vi "Loading sci QT.vi"(0 "Absolute start time (ms)":dbl=51099.288 format="%.3f", 1 "Static input":T4(array[cluster])=[{"Times"=[6954.0, 7000.1], "Voltages"=[-0.1, -1.0], "Enable Ch"=TRUE, "Hinge Points"=2}, {"Times"=[6944.0, 6994.0, 7000.0], "Voltages"=[-1.0, 2.5, -1.0], "Enable Ch"=TRUE, "Hinge Points"=3}, {"Times"=[6944.0, 6994.0, 7000.0], "Voltages"=[0.0, 0.6, -1.0], "Enable Ch"=TRUE, "Hinge Points"=3}, {"Times"=[6944.0, 6994.0, 7000.0], "Voltages"=[4.0, 0.65, -1.0], "Enable Ch"=TRUE, "Hinge Points"=3}, {"Times"=[6992.0, 7000.6], "Voltages"=[0.0, 2.7], "Enable Ch"=TRUE, "Hinge Points"=2}, {"Times"=[7000.6, 7011.1], "Voltages"=[0.25, 3.0], "Enable Ch"=TRUE, "Hinge Points"=2}, {"Times"=[], "Voltages"=[], "Enable Ch"=TRUE, "Hinge Points"=0}, {"Times"=[48001.288, 48011.488, 48021.688, 48031.888, 48042.088, 48052.288, 48062.488, 48072.688, 48082.888, 48093.088, 48103.288, 48113.488, 48123.688, 48133.888, 48144.088, 48154.288, 48164.488, 48174.688, 48184.888, 48195.088, 48205.288, 48215.488, 48225.688, 48235.888, 48246.088, 48256.288, 48266.488, 48276.688, 48286.888, 48297.088, 48307.288, 48317.488, 48327.688, 48337.888, 48348.088, 48358.288, 48368.488, 48378.688, 48388.888, 48399.088, 48409.288, 48419.488, 48429.688, 48439.888, 48450.088, 48460.288, 48470.488, 48480.688, 48490.888, 48501.088, 48511.288], "Voltages"=[0.0, -0.0052, -0.0104, -0.0156, -0.0208, -0.026, -0.0312, -0.0364, -0.0416, -0.046799999999999994, -0.052, -0.0572, -0.0624, -0.0676, -0.0728, -0.078, -0.0832, -0.08839999999999999, -0.09359999999999999, -0.0988, -0.104, -0.10919999999999999, -0.1144, -0.1196, -0.1248, -0.13, -0.1352, -0.1404, -0.1456, -0.1508, -0.156, -0.16119999999999998, -0.1664, -0.1716, -0.17679999999999998, -0.182, -0.18719999999999998, -0.1924, -0.1976, -0.20279999999999998, -0.208, -0.2132, -0.21839999999999998, -0.2236, -0.2288, -0.23399999999999999, -0.2392, -0.24439999999999998, -0.2496, -0.25479999999999997, -0.26], "Enable Ch"=TRUE, "Hinge Points"=51}, {"Times"=[6944.0, 6994.0, 7000.1, 7004.1, 47301.288, 47631.288, 50900.288, 51105.288], "Voltages"=[0.1635, 0.12, -0.63, 0.0, 0.067, -0.004, 1.44, -0.004], "Enable Ch"=TRUE, "Hinge Points"=8}, {"Times"=[6994.0, 7000.0, 7001.0, 7003.1, 7103.1, 7105.6, 7108.1, 7110.6, 7113.1, 7115.6, 7118.1, 7120.6, 7123.1, 7125.6, 7128.1, 7130.6, 7133.1, 7135.6, 7138.1, 7140.6, 7143.1, 7145.6, 7148.1, 7150.6, 7153.1, 7155.6, 7158.1, 7160.6, 7163.1, 7165.6, 7168.1, 7170.6, 7173.1, 7175.6, 7178.1, 7180.6, 7183.1, 7185.6, 7188.1, 7190.6, 7193.1, 7195.6, 7198.1, 7200.6, 7203.1, 7205.6, 7208.1, 7210.6, 7213.1, 7215.6, 7218.1, 7220.6, 7223.1, 7225.6, 7228.1, 7230.6, 7233.1, 7235.6, 7238.1, 7240.6, 7243.1, 7245.6, 7248.1, 7250.6, 7253.1, 7255.6, 7258.1, 7260.6, 7263.1, 7265.6, 7268.1, 7270.6, 7273.1, 7275.6, 7278.1, 7280.6, 7283.1, 7285.6, 7288.1, 7290.6, 7293.1, 7295.6, 7298.1, 7300.6, 7303.1, 7305.6, 7308.1, 7310.6, 7313.1, 7315.6, 7318.1, 7320.6, 7323.1, 7325.6, 7328.1, 7330.6, 7333.1, 7335.6, 7338.1, 7340.6, 7343.1, 7345.6, 7348.1, 7350.6, 7353.1, 10849.9], "Voltages"=[-1.0, -10.0, 0.0, 1.8, 1.8, 1.854, 1.9080000000000001, 1.9620000000000002, 2.016, 2.0700000000000003, 2.124, 2.178, 2.232, 2.286, 2.34, 2.394, 2.4480000000000004, 2.5020000000000002, 2.556, 2.6100000000000003, 2.664, 2.718, 2.7720000000000002, 2.826, 2.88, 2.934, 2.9880000000000004, 3.0420000000000003, 3.096, 3.1500000000000004, 3.204, 3.258, 3.3120000000000003, 3.3660000000000005, 3.42, 3.474, 3.5280000000000005, 3.5820000000000003, 3.636, 3.6900000000000004, 3.744, 3.798, 3.8520000000000003, 3.9060000000000006, 3.96, 4.014, 4.0680000000000005, 4.122, 4.176, 4.23, 4.284000000000001, 4.338, 4.392, 4.446000000000001, 4.5, 4.554, 4.6080000000000005, 4.662000000000001, 4.716, 4.7700000000000005, 4.824000000000001, 4.878, 4.932, 4.986000000000001, 5.04, 5.094, 5.148000000000001, 5.202000000000001, 5.256, 5.3100000000000005, 5.364000000000001, 5.418, 5.472, 5.526000000000001, 5.58, 5.634, 5.688000000000001, 5.742000000000001, 5.796, 5.8500000000000005, 5.904, 5.958, 6.0120000000000005, 6.066000000000001, 6.12, 6.174, 6.228000000000001, 6.282, 6.336, 6.390000000000001, 6.444, 6.498, 6.5520000000000005, 6.606000000000001, 6.66, 6.714, 6.768000000000001, 6.822, 6.876, 6.930000000000001, 6.984000000000001, 7.038, 7.0920000000000005, 7.146000000000001, 7.2, -1.0], "Enable Ch"=TRUE, "Hinge Points"=106}, {"Times"=[7001.0, 6978.1, 7008.1, 7093.1, 7095.6, 7098.1, 7100.6, 7103.1, 7105.6, 7108.1, 7110.6, 7113.1, 7115.6, 7118.1, 7120.6, 7123.1, 7125.6, 7128.1, 7130.6, 7133.1, 7135.6, 7138.1, 7140.6, 7143.1, 7145.6, 7148.1, 7150.6, 7153.1, 7155.6, 7158.1, 7160.6, 7163.1, 7165.6, 7168.1, 7170.6, 7173.1, 7175.6, 7178.1, 7180.6, 7183.1, 7185.6, 7188.1, 7190.6, 7193.1, 7195.6, 7198.1, 7200.6, 7203.1, 7205.6, 7208.1, 7210.6, 7213.1, 7215.6, 7218.1, 7220.6, 7223.1, 7225.6, 7228.1, 7230.6, 7233.1, 7235.6, 7238.1, 7240.6, 7243.1, 7245.6, 7248.1, 7250.6, 7253.1, 7255.6, 7258.1, 7260.6, 7263.1, 7265.6, 7268.1, 7270.6, 7273.1, 7275.6, 7278.1, 7280.6, 7283.1, 7285.6, 7288.1, 7290.6, 7293.1, 7295.6, 7298.1, 7300.6, 7303.1, 7305.6, 7308.1, 7310.6, 7313.1, 7315.6, 7318.1, 7320.6, 7323.1, 7325.6, 7328.1, 7330.6, 7333.1, 7335.6, 7338.1, 7340.6, 7343.1, 10855.0, 47201.288, 47206.288, 47951.288, 48101.788, 48471.288], "Voltages"=[-0.4, -2.5, -0.78, -0.78, -0.8009000000000001, -0.8218, -0.8427, -0.8636, -0.8845000000000001, -0.9054, -0.9263, -0.9472, -0.9681, -0.989, -1.0099, -1.0308, -1.0517, -1.0726, -1.0935000000000001, -1.1144, -1.1353, -1.1562000000000001, -1.1771, -1.198, -1.2189, -1.2398, -1.2607, -1.2816, -1.3025, -1.3234, -1.3443, -1.3652, -1.3860999999999999, -1.407, -1.4279, -1.4487999999999999, -1.4697, -1.4906, -1.5114999999999998, -1.5324, -1.5533000000000001, -1.5741999999999998, -1.5951, -1.616, -1.6368999999999998, -1.6578, -1.6787, -1.6996, -1.7205, -1.7414, -1.7623, -1.7832, -1.8041, -1.825, -1.8458999999999999, -1.8668, -1.8877, -1.9085999999999999, -1.9295, -1.9504, -1.9712999999999998, -1.9922, -2.0130999999999997, -2.034, -2.0549, -2.0758, -2.0967000000000002, -2.1176, -2.1384999999999996, -2.1593999999999998, -2.1803, -2.2012, -2.2221, -2.243, -2.2639, -2.2847999999999997, -2.3057, -2.3266, -2.3475, -2.3684, -2.3893, -2.4101999999999997, -2.4311, -2.452, -2.4729, -2.4938, -2.5147, -2.5355999999999996, -2.5564999999999998, -2.5774, -2.5983, -2.6192, -2.6401, -2.6609999999999996, -2.6818999999999997, -2.7028, -2.7237, -2.7446, -2.7655, -2.7863999999999995, -2.8072999999999997, -2.8282, -2.8491, -2.87, -1.52, -0.5, -0.15, -2.0, -1.8, -2.4], "Enable Ch"=TRUE, "Hinge Points"=110}, {"Times"=[6944.0, 6994.0, 7000.6], "Voltages"=[0.15, 0.2, 2.5], "Enable Ch"=TRUE, "Hinge Points"=3}, {"Times"=[10850.0, 47200.188, 47200.288, 47200.338, 47200.388, 47200.438, 47200.488, 47200.538, 47200.588, 47200.638, 47200.688, 47200.738, 47200.788, 47200.838, 47200.888, 47200.938, 47200.988, 47201.038, 47201.088, 47201.138, 47201.188, 47201.238, 47201.288, 48501.788, 48001.288, 48003.788, 48006.288, 48008.788, 48011.288, 48013.788, 48016.288, 48018.788, 48021.288, 48023.788, 48026.288, 48028.788, 48031.288, 48033.788, 48036.288, 48038.788, 48041.288, 48043.788, 48046.288, 48048.788, 48051.288, 48053.788, 48056.288, 48058.788, 48061.288, 48063.788, 48066.288, 48068.788, 48071.288, 48073.788, 48076.288, 48078.788, 48081.288, 48083.788, 48086.288, 48088.788, 48091.288, 48093.788, 48096.288, 48098.788, 48101.288, 48103.788, 48106.288, 48108.788, 48111.288, 48113.788, 48116.288, 48118.788, 48121.288, 48123.788, 48126.288, 48128.788, 48131.288, 48133.788, 48136.288, 48138.788, 48141.288, 48143.788, 48146.288, 48148.788, 48151.288, 48153.788, 48156.288, 48158.788, 48161.288, 48163.788, 48166.288, 48168.788, 48171.288, 48173.788, 48176.288, 48178.788, 48181.288, 48183.788, 48186.288, 48188.788, 48191.288, 48193.788, 48196.288, 48198.788, 48201.288, 48203.788, 48206.288, 48208.788, 48211.288, 48213.788, 48216.288, 48218.788, 48221.288, 48223.788, 48226.288, 48228.788, 48231.288, 48233.788, 48236.288, 48238.788, 48241.288, 48243.788, 48246.288, 48248.788, 48251.288, 48253.788, 48256.288, 48258.788, 48261.288, 48263.788, 48266.288, 48268.788, 48271.288, 48273.788, 48276.288, 48278.788, 48281.288, 48283.788, 48286.288, 48288.788, 48291.288, 48293.788, 48296.288, 48298.788, 48301.288, 48303.788, 48306.288, 48308.788, 48311.288, 48313.788, 48316.288, 48318.788, 48321.288, 48323.788, 48326.288, 48328.788, 48331.288, 48333.788, 48336.288, 48338.788, 48341.288, 48343.788, 48346.288, 48348.788, 48351.288, 48353.788, 48356.288, 48358.788, 48361.288, 48363.788, 48366.288, 48368.788, 48371.288, 48373.788, 48376.288, 48378.788, 48381.288, 48383.788, 48386.288, 48388.788, 48391.288, 48393.788, 48396.288, 48398.788, 48401.288, 48403.788, 48406.288, 48408.788, 48411.288, 48413.788, 48416.288, 48418.788, 48421.288, 48423.788, 48426.288, 48428.788, 48431.288, 48433.788, 48436.288, 48438.788, 48441.288, 48443.788, 48446.288, 48448.788, 48451.288, 48453.788, 48456.288, 48458.788, 48461.288, 48463.788, 48466.288, 48468.788, 48471.288, 48473.788, 48476.288, 48478.788, 48481.288, 48483.788, 48486.288, 48488.788, 48491.288, 48493.788, 48496.288, 48498.788, 48501.288], "Voltages"=[0.0, 2.978, 2.978, 2.8241, 2.6702000000000004, 2.5163, 2.3624, 2.2085, 2.0546, 1.9007, 1.7468000000000001, 1.5929000000000002, 1.439, 1.2851000000000001, 1.1312000000000002, 0.9773000000000001, 0.8233999999999999, 0.6695000000000002, 0.5156000000000001, 0.3616999999999999, 0.2078000000000002, 0.05390000000000006, -0.10000000000000009, 0.0, 0.0, 0.00065, 0.0013, 0.00195, 0.0026, 0.00325, 0.0039, 0.00455, 0.0052, 0.005849999999999999, 0.0065, 0.00715, 0.0078, 0.00845, 0.0091, 0.00975, 0.0104, 0.011049999999999999, 0.011699999999999999, 0.01235, 0.013, 0.013649999999999999, 0.0143, 0.01495, 0.0156, 0.01625, 0.0169, 0.01755, 0.0182, 0.01885, 0.0195, 0.020149999999999998, 0.0208, 0.02145, 0.022099999999999998, 0.02275, 0.023399999999999997, 0.02405, 0.0247, 0.025349999999999998, 0.026, 0.02665, 0.027299999999999998, 0.02795, 0.0286, 0.029249999999999998, 0.0299, 0.030549999999999997, 0.0312, 0.031849999999999996, 0.0325, 0.03315, 0.0338, 0.03445, 0.0351, 0.03575, 0.0364, 0.03705, 0.0377, 0.038349999999999995, 0.039, 0.03965, 0.040299999999999996, 0.04095, 0.0416, 0.042249999999999996, 0.0429, 0.04355, 0.044199999999999996, 0.04485, 0.0455, 0.04615, 0.046799999999999994, 0.04745, 0.0481, 0.048749999999999995, 0.0494, 0.05005, 0.050699999999999995, 0.05135, 0.052, 0.052649999999999995, 0.0533, 0.05395, 0.054599999999999996, 0.05525, 0.0559, 0.056549999999999996, 0.0572, 0.05785, 0.058499999999999996, 0.059149999999999994, 0.0598, 0.06045, 0.061099999999999995, 0.06175, 0.0624, 0.06305, 0.06369999999999999, 0.06434999999999999, 0.065, 0.06565, 0.0663, 0.06695, 0.0676, 0.06824999999999999, 0.0689, 0.06955, 0.0702, 0.07085, 0.0715, 0.07214999999999999, 0.0728, 0.07345, 0.0741, 0.07475, 0.0754, 0.07604999999999999, 0.07669999999999999, 0.07735, 0.078, 0.07865, 0.0793, 0.07995, 0.08059999999999999, 0.08125, 0.0819, 0.08255, 0.0832, 0.08385, 0.08449999999999999, 0.08514999999999999, 0.0858, 0.08645, 0.0871, 0.08775, 0.08839999999999999, 0.08904999999999999, 0.0897, 0.09035, 0.091, 0.09165, 0.0923, 0.09294999999999999, 0.09359999999999999, 0.09425, 0.0949, 0.09555, 0.0962, 0.09684999999999999, 0.09749999999999999, 0.09815, 0.0988, 0.09945, 0.1001, 0.10074999999999999, 0.10139999999999999, 0.10205, 0.1027, 0.10335, 0.104, 0.10464999999999999, 0.10529999999999999, 0.10594999999999999, 0.1066, 0.10725, 0.1079, 0.10855, 0.10919999999999999, 0.10984999999999999, 0.1105, 0.11115, 0.1118, 0.11245, 0.11309999999999999, 0.11374999999999999, 0.1144, 0.11505, 0.1157, 0.11635, 0.11699999999999999, 0.11764999999999999, 0.11829999999999999, 0.11895, 0.1196, 0.12025, 0.1209, 0.12154999999999999, 0.12219999999999999, 0.12285, 0.1235, 0.12415, 0.1248, 0.12545, 0.1261, 0.12675, 0.12739999999999999, 0.12805, 0.12869999999999998, 0.12935, 0.13], "Enable Ch"=TRUE, "Hinge Points"=225}, {"Times"=[10850.0, 10950.0, 10959.0, 10968.0, 10977.0, 10986.0, 10995.0, 11004.0, 11013.0, 11022.0, 11031.0, 11040.0, 11049.0, 11058.0, 11067.0, 11076.0, 11085.0, 11094.0, 11103.0, 11112.0, 11121.0, 11130.0, 11139.0, 11148.0, 11157.0, 11166.0, 11175.0, 11184.0, 11193.0, 11202.0, 11211.0, 11220.0, 11229.0, 11238.0, 11247.0, 11256.0, 11265.0, 11274.0, 11283.0, 11292.0, 11301.0, 11310.0, 11319.0, 11328.0, 11337.0, 11346.0, 11355.0, 11364.0, 11373.0, 11382.0, 11391.0, 11400.0, 11409.0, 11418.0, 11427.0, 11436.0, 11445.0, 11454.0, 11463.0, 11472.0, 11481.0, 11490.0, 11499.0, 11508.0, 11517.0, 11526.0, 11535.0, 11544.0, 11553.0, 11562.0, 11571.0, 11580.0, 11589.0, 11598.0, 11607.0, 11616.0, 11625.0, 11634.0, 11643.0, 11652.0, 11661.0, 11670.0, 11679.0, 11688.0, 11697.0, 11706.0, 11715.0, 11724.0, 11733.0, 11742.0, 11751.0, 11760.0, 11769.0, 11778.0, 11787.0, 11796.0, 11805.0, 11814.0, 11823.0, 11832.0, 11841.0, 11850.0, 47191.188, 47200.288, 47205.288, 47201.288, 47201.338, 47201.388, 47201.438, 47201.488, 47201.538, 47201.588, 47201.638, 47201.688, 47201.738, 47201.788, 47201.838, 47201.888, 47201.938, 47201.988, 47202.038, 47202.088, 47202.138, 47202.188, 47202.238, 47202.288, 47202.338, 47202.388, 47202.438, 47202.488, 47202.538, 47202.588, 47202.638, 47202.688, 47202.738, 47202.788, 47202.838, 47202.888, 47202.938, 47202.988, 47203.038, 47203.088, 47203.138, 47203.188, 47203.238, 47203.288, 47203.338, 47203.388, 47203.438, 47203.488, 47203.538, 47203.588, 47203.638, 47203.688, 47203.738, 47203.788, 47203.838, 47203.888, 47203.938, 47203.988, 47204.038, 47204.088, 47204.138, 47204.188, 47204.238, 47204.288, 47191.288, 47191.348, 47191.408, 47191.468, 47191.528, 47191.588, 47191.648, 47191.708, 47191.768000000004, 47191.828, 47191.888, 47191.948000000004, 47192.008, 47192.068, 47192.128, 47192.188, 47192.248, 47192.308, 47192.368, 47192.428, 47192.488, 47192.548, 47192.608, 47192.668, 47192.728, 47192.788, 47192.848, 47192.908, 47192.968, 47193.028, 47193.088, 47193.148, 47193.208, 47193.268000000004, 47193.328, 47193.388, 47193.448000000004, 47193.508, 47193.568, 47193.628, 47193.688, 47193.748, 47193.808, 47193.868, 47193.928, 47193.988, 47194.048, 47194.108, 47194.168, 47194.228, 47194.288, 47194.348, 47194.408, 47194.468, 47194.528, 47194.588, 47194.648, 47194.708, 47194.768000000004, 47194.828, 47194.888, 47194.948000000004, 47195.008, 47195.068, 47195.128, 47195.188, 47195.248, 47195.308, 47195.368, 47195.428, 47195.488, 47195.548, 47195.608, 47195.668, 47195.728, 47195.788, 47195.848, 47195.908, 47195.968, 47196.028, 47196.088, 47196.148, 47196.208, 47196.268000000004, 47196.328, 47196.388, 47196.448000000004, 47196.508, 47196.568, 47196.628, 47196.688, 47196.748, 47196.808, 47196.868, 47196.928, 47196.988, 47197.048, 47197.108, 47197.168, 47197.228, 47197.288, 47501.288, 47501.288, 47501.368, 47501.448000000004, 47501.528, 47501.608, 47501.688, 47501.768000000004, 47501.848, 47501.928, 47502.008, 47502.088, 47502.168, 47502.248, 47502.328, 47502.408, 47502.488, 47502.568, 47502.648, 47502.728, 47502.808, 47502.888, 47502.968, 47503.048, 47503.128, 47503.208, 47503.288, 47503.368, 47503.448000000004, 47503.528, 47503.608, 47503.688, 47503.768000000004, 47503.848, 47503.928, 47504.008, 47504.088, 47504.168, 47504.248, 47504.328, 47504.408, 47504.488, 47504.568, 47504.648, 47504.728, 47504.808, 47504.888, 47504.968, 47505.048, 47505.128, 47505.208, 47505.288, 48511.788, 48001.288, 48003.788, 48006.288, 48008.788, 48011.288, 48013.788, 48016.288, 48018.788, 48021.288, 48023.788, 48026.288, 48028.788, 48031.288, 48033.788, 48036.288, 48038.788, 48041.288, 48043.788, 48046.288, 48048.788, 48051.288, 48053.788, 48056.288, 48058.788, 48061.288, 48063.788, 48066.288, 48068.788, 48071.288, 48073.788, 48076.288, 48078.788, 48081.288, 48083.788, 48086.288, 48088.788, 48091.288, 48093.788, 48096.288, 48098.788, 48101.288, 48103.788, 48106.288, 48108.788, 48111.288, 48113.788, 48116.288, 48118.788, 48121.288, 48123.788, 48126.288, 48128.788, 48131.288, 48133.788, 48136.288, 48138.788, 48141.288, 48143.788, 48146.288, 48148.788, 48151.288, 48153.788, 48156.288, 48158.788, 48161.288, 48163.788, 48166.288, 48168.788, 48171.288, 48173.788, 48176.288, 48178.788, 48181.288, 48183.788, 48186.288, 48188.788, 48191.288, 48193.788, 48196.288, 48198.788, 48201.288, 48203.788, 48206.288, 48208.788, 48211.288, 48213.788, 48216.288, 48218.788, 48221.288, 48223.788, 48226.288, 48228.788, 48231.288, 48233.788, 48236.288, 48238.788, 48241.288, 48243.788, 48246.288, 48248.788, 48251.288, 48253.788, 48256.288, 48258.788, 48261.288, 48263.788, 48266.288, 48268.788, 48271.288, 48273.788, 48276.288, 48278.788, 48281.288, 48283.788, 48286.288, 48288.788, 48291.288, 48293.788, 48296.288, 48298.788, 48301.288, 48303.788, 48306.288, 48308.788, 48311.288, 48313.788, 48316.288, 48318.788, 48321.288, 48323.788, 48326.288, 48328.788, 48331.288, 48333.788, 48336.288, 48338.788, 48341.288, 48343.788, 48346.288, 48348.788, 48351.288, 48353.788, 48356.288, 48358.788, 48361.288, 48363.788, 48366.288, 48368.788, 48371.288, 48373.788, 48376.288, 48378.788, 48381.288, 48383.788, 48386.288, 48388.788, 48391.288, 48393.788, 48396.288, 48398.788, 48401.288, 48403.788, 48406.288, 48408.788, 48411.288, 48413.788, 48416.288, 48418.788, 48421.288, 48423.788, 48426.288, 48428.788, 48431.288, 48433.788, 48436.288, 48438.788, 48441.288, 48443.788, 48446.288, 48448.788, 48451.288, 48453.788, 48456.288, 48458.788, 48461.288, 48463.788, 48466.288, 48468.788, 48471.288, 48473.788, 48476.288, 48478.788, 48481.288, 48483.788, 48486.288, 48488.788, 48491.288, 48493.788, 48496.288, 48498.788, 48501.288, 48501.288, 48502.288, 48503.288, 48504.288, 48505.288, 48506.288, 48507.288, 48508.288, 48509.288, 48510.288, 48511.288, 50899.288, 50904.288, 50909.288, 50914.288, 50919.288, 50924.288, 50929.288, 50934.288, 50939.288, 50944.288, 50949.288, 50954.288, 50959.288, 50964.288, 50969.288, 50974.288, 50979.288, 50984.288, 50989.288, 50994.288, 50999.288, 51098.288, 51098.29466666667, 51098.30133333334, 51098.308, 51098.314666666665, 51098.32133333333, 51098.328, 51098.33466666667, 51098.34133333334, 51098.348, 51098.354666666666, 51098.361333333334, 51098.368, 51098.37466666667, 51098.38133333333, 51098.388, 51098.39466666667, 51098.401333333335, 51098.408, 51098.414666666664, 51098.42133333333, 51098.428, 51098.43466666667, 51098.441333333336, 51098.448000000004, 51098.454666666665, 51098.46133333333, 51098.468, 51098.47466666667, 51098.48133333334, 51098.488, 51098.494666666666, 51098.50133333333, 51098.508, 51098.51466666667, 51098.52133333333, 51098.528, 51098.53466666667, 51098.541333333334, 51098.548, 51098.55466666667, 51098.56133333333, 51098.568, 51098.57466666667, 51098.581333333335, 51098.588, 51098.594666666664, 51098.60133333333, 51098.608, 51098.61466666667, 51098.621333333336, 51098.628, 51098.634666666665, 51098.64133333333, 51098.648, 51098.65466666667, 51098.66133333334, 51098.668, 51098.674666666666, 51098.681333333334, 51098.688, 51098.69466666667, 51098.70133333333, 51098.708, 51098.71466666667, 51098.721333333335, 51098.728, 51098.73466666666, 51098.74133333333, 51098.748, 51098.75466666667, 51098.761333333336, 51098.768000000004, 51098.774666666664, 51098.78133333333, 51098.788, 51098.79466666667, 51098.80133333334, 51098.808, 51098.814666666665, 51098.82133333333, 51098.828, 51098.83466666667, 51098.84133333334, 51098.848, 51098.854666666666, 51098.861333333334, 51098.868, 51098.87466666667, 51098.88133333333, 51098.888, 51098.89466666667, 51098.901333333335, 51098.908, 51098.914666666664, 51098.92133333333, 51098.928, 51098.93466666667, 51098.941333333336, 51098.948000000004, 51098.954666666665, 51098.96133333333, 51098.968, 51098.97466666667, 51098.98133333334, 51098.988, 51098.994666666666, 51099.00133333333, 51099.008, 51099.01466666667, 51099.02133333333, 51099.028, 51099.03466666667, 51099.041333333334, 51099.048, 51099.05466666667, 51099.06133333333, 51099.068, 51099.07466666667, 51099.081333333335, 51099.088, 51099.094666666664, 51099.10133333333, 51099.108, 51099.11466666667, 51099.121333333336, 51099.128, 51099.134666666665, 51099.14133333333, 51099.148, 51099.15466666667, 51099.16133333334, 51099.168, 51099.174666666666, 51099.181333333334, 51099.188, 51099.19466666667, 51099.20133333333, 51099.208, 51099.21466666667, 51099.221333333335, 51099.228, 51099.23466666666, 51099.24133333333, 51099.248, 51099.25466666667, 51099.261333333336, 51099.268000000004, 51099.274666666664, 51099.28133333333, 51099.288], "Voltages"=[0.8, 0.8, 0.803575, 0.80715, 0.810725, 0.8143, 0.817875, 0.82145, 0.825025, 0.8286, 0.832175, 0.83575, 0.839325, 0.8429, 0.8464750000000001, 0.8500500000000001, 0.8536250000000001, 0.8572000000000001, 0.8607750000000001, 0.8643500000000001, 0.8679250000000001, 0.8715, 0.875075, 0.87865, 0.882225, 0.8858, 0.889375, 0.89295, 0.896525, 0.9001, 0.903675, 0.90725, 0.910825, 0.9144, 0.917975, 0.92155, 0.925125, 0.9287000000000001, 0.932275, 0.9358500000000001, 0.939425, 0.9430000000000001, 0.9465749999999999, 0.95015, 0.953725, 0.9573, 0.960875, 0.96445, 0.968025, 0.9716, 0.975175, 0.97875, 0.982325, 0.9859, 0.989475, 0.99305, 0.996625, 1.0002, 1.003775, 1.00735, 1.010925, 1.0145, 1.018075, 1.02165, 1.025225, 1.0288, 1.032375, 1.03595, 1.039525, 1.0431, 1.046675, 1.05025, 1.053825, 1.0574, 1.060975, 1.06455, 1.068125, 1.0716999999999999, 1.075275, 1.07885, 1.082425, 1.0859999999999999, 1.089575, 1.09315, 1.096725, 1.1003, 1.103875, 1.10745, 1.111025, 1.1146, 1.118175, 1.12175, 1.125325, 1.1289, 1.132475, 1.13605, 1.1396249999999999, 1.1432, 1.1467749999999999, 1.15035, 1.153925, 1.1575, 1.15, 0.0, 0.0, 0.0, 0.004699999999999999, 0.009399999999999999, 0.014099999999999998, 0.018799999999999997, 0.023499999999999997, 0.028199999999999996, 0.0329, 0.037599999999999995, 0.04229999999999999, 0.04699999999999999, 0.051699999999999996, 0.05639999999999999, 0.06109999999999999, 0.0658, 0.0705, 0.07519999999999999, 0.07989999999999998, 0.08459999999999998, 0.08929999999999999, 0.09399999999999999, 0.09869999999999998, 0.10339999999999999, 0.10809999999999999, 0.11279999999999998, 0.11749999999999998, 0.12219999999999998, 0.12689999999999999, 0.1316, 0.13629999999999998, 0.141, 0.14569999999999997, 0.15039999999999998, 0.1551, 0.15979999999999997, 0.16449999999999998, 0.16919999999999996, 0.17389999999999997, 0.17859999999999998, 0.18329999999999996, 0.18799999999999997, 0.19269999999999998, 0.19739999999999996, 0.20209999999999997, 0.20679999999999998, 0.21149999999999997, 0.21619999999999998, 0.22089999999999996, 0.22559999999999997, 0.23029999999999998, 0.23499999999999996, 0.23969999999999997, 0.24439999999999995, 0.24909999999999996, 0.25379999999999997, 0.25849999999999995, 0.2632, 0.26789999999999997, 0.27259999999999995, 0.27729999999999994, 0.282, 1.15, 1.13852, 1.1270399999999998, 1.1155599999999999, 1.10408, 1.0926, 1.0811199999999999, 1.06964, 1.05816, 1.0466799999999998, 1.0352, 1.02372, 1.0122399999999998, 1.0007599999999999, 0.9892799999999999, 0.9777999999999999, 0.96632, 0.9548399999999999, 0.94336, 0.9318799999999999, 0.9203999999999999, 0.90892, 0.89744, 0.8859599999999999, 0.8744799999999999, 0.863, 0.8515199999999999, 0.8400399999999999, 0.82856, 0.8170799999999999, 0.8055999999999999, 0.7941199999999999, 0.78264, 0.77116, 0.7596799999999999, 0.7482, 0.7367199999999999, 0.7252399999999999, 0.71376, 0.70228, 0.6908, 0.6793199999999999, 0.66784, 0.6563599999999999, 0.64488, 0.6334, 0.6219199999999999, 0.61044, 0.5989599999999999, 0.58748, 0.576, 0.56452, 0.55304, 0.5415599999999999, 0.53008, 0.5186, 0.50712, 0.49563999999999997, 0.4841599999999999, 0.47268, 0.46119999999999994, 0.44972, 0.43823999999999996, 0.42676000000000003, 0.41528, 0.40379999999999994, 0.39232, 0.38083999999999996, 0.36936, 0.35788, 0.34640000000000004, 0.33492, 0.32343999999999995, 0.31196, 0.30047999999999997, 0.28900000000000003, 0.27752, 0.26603999999999994, 0.25456, 0.24307999999999996, 0.23160000000000003, 0.22011999999999998, 0.20864000000000005, 0.19716, 0.18567999999999996, 0.17420000000000002, 0.16271999999999998, 0.15124000000000004, 0.1397600000000001, 0.12827999999999995, 0.11680000000000001, 0.10532000000000008, 0.09383999999999992, 0.08235999999999999, 0.07088000000000005, 0.05940000000000012, 0.04791999999999996, 0.03644000000000003, 0.024960000000000093, 0.013479999999999936, 0.0020000000000000018, 0.282, 0.282, 0.27727999999999997, 0.27255999999999997, 0.26783999999999997, 0.26311999999999997, 0.25839999999999996, 0.25367999999999996, 0.24896, 0.24423999999999998, 0.23951999999999998, 0.23479999999999998, 0.23007999999999998, 0.22535999999999998, 0.22063999999999998, 0.21592, 0.2112, 0.20648, 0.20176, 0.19704, 0.19232, 0.1876, 0.18288, 0.17815999999999999, 0.17343999999999998, 0.16871999999999998, 0.16399999999999998, 0.15927999999999998, 0.15456, 0.14984, 0.14512, 0.1404, 0.13568, 0.13096, 0.12624, 0.12151999999999999, 0.11679999999999999, 0.11207999999999999, 0.10735999999999998, 0.10264000000000001, 0.09792000000000001, 0.0932, 0.08848, 0.08376, 0.07904, 0.07432, 0.0696, 0.06488, 0.06015999999999999, 0.05543999999999999, 0.050720000000000015, 0.04600000000000001, -1.86, 0.046, 0.06577, 0.08554, 0.10531, 0.12508, 0.14484999999999998, 0.16462, 0.18439, 0.20416, 0.22393000000000002, 0.24369999999999997, 0.26347, 0.28324, 0.30301, 0.32277999999999996, 0.34254999999999997, 0.36232, 0.38209, 0.40186, 0.42162999999999995, 0.44139999999999996, 0.46116999999999997, 0.48094, 0.50071, 0.52048, 0.54025, 0.5600200000000001, 0.57979, 0.59956, 0.61933, 0.6391, 0.6588700000000001, 0.67864, 0.69841, 0.71818, 0.73795, 0.7577200000000001, 0.77749, 0.79726, 0.81703, 0.8368, 0.85657, 0.87634, 0.89611, 0.91588, 0.93565, 0.95542, 0.97519, 0.9949600000000001, 1.01473, 1.0345, 1.05427, 1.07404, 1.09381, 1.11358, 1.13335, 1.15312, 1.17289, 1.19266, 1.21243, 1.2322, 1.25197, 1.27174, 1.29151, 1.31128, 1.33105, 1.35082, 1.37059, 1.39036, 1.41013, 1.4299, 1.44967, 1.46944, 1.48921, 1.50898, 1.52875, 1.54852, 1.56829, 1.58806, 1.60783, 1.6276, 1.64737, 1.66714, 1.68691, 1.70668, 1.72645, 1.7462199999999999, 1.76599, 1.78576, 1.80553, 1.8253, 1.84507, 1.86484, 1.88461, 1.90438, 1.92415, 1.94392, 1.96369, 1.98346, 2.00323, 2.0229999999999997, 2.04277, 2.06254, 2.0823099999999997, 2.10208, 2.12185, 2.1416199999999996, 2.16139, 2.1811599999999998, 2.2009299999999996, 2.2207, 2.2404699999999997, 2.2602399999999996, 2.28001, 2.2997799999999997, 2.3195499999999996, 2.33932, 2.3590899999999997, 2.3788599999999995, 2.39863, 2.4183999999999997, 2.43817, 2.45794, 2.4777099999999996, 2.49748, 2.5172499999999998, 2.5370199999999996, 2.55679, 2.5765599999999997, 2.5963299999999996, 2.6161, 2.6358699999999997, 2.6556399999999996, 2.67541, 2.6951799999999997, 2.7149499999999995, 2.73472, 2.7544899999999997, 2.77426, 2.79403, 2.8137999999999996, 2.83357, 2.8533399999999998, 2.8731099999999996, 2.89288, 2.9126499999999997, 2.9324199999999996, 2.95219, 2.9719599999999997, 2.9917299999999996, 3.0115, 3.0312699999999997, 3.0510399999999995, 3.07081, 3.0905799999999997, 3.1103499999999995, 3.13012, 3.1498899999999996, 3.16966, 3.1894299999999998, 3.2091999999999996, 3.22897, 3.2487399999999997, 3.2685099999999996, 3.28828, 3.3080499999999997, 3.3278199999999996, 3.34759, 3.3673599999999997, 3.3871299999999995, 3.4069, 3.4266699999999997, 3.4464399999999995, 3.46621, 3.4859799999999996, 3.50575, 3.5255199999999998, 3.5452899999999996, 3.56506, 3.5848299999999997, 3.6045999999999996, 3.62437, 3.6441399999999997, 3.6639099999999996, 3.68368, 3.7034499999999997, 3.7232199999999995, 3.74299, 3.7627599999999997, 3.7825299999999995, 3.8023, 3.8220699999999996, 3.84184, 3.8616099999999998, 3.8813799999999996, 3.90115, 3.9209199999999997, 3.9406899999999996, 3.96046, 3.9802299999999997, 3.9999999999999996, 4.0, 4.092, 4.184, 4.276, 4.368, 4.46, 4.552, 4.644, 4.736, 4.828, 4.92, -1.86, -1.9432500000000001, -2.0265, -2.10975, -2.193, -2.27625, -2.3595, -2.44275, -2.526, -2.6092500000000003, -2.6925, -2.77575, -2.859, -2.94225, -3.0255, -3.1087499999999997, -3.192, -3.2752499999999998, -3.3585000000000003, -3.44175, -3.525, -3.525, -3.5307666666666666, -3.5365333333333333, -3.5423, -3.5480666666666667, -3.5538333333333334, -3.5596, -3.5653666666666664, -3.571133333333333, -3.5768999999999997, -3.5826666666666664, -3.588433333333333, -3.5942, -3.5999666666666665, -3.6057333333333332, -3.6115, -3.6172666666666666, -3.6230333333333333, -3.6288, -3.6345666666666667, -3.6403333333333334, -3.6460999999999997, -3.6518666666666664, -3.657633333333333, -3.6633999999999998, -3.6691666666666665, -3.674933333333333, -3.6807, -3.6864666666666666, -3.6922333333333333, -3.698, -3.7037666666666667, -3.7095333333333333, -3.7153, -3.7210666666666663, -3.726833333333333, -3.7325999999999997, -3.7383666666666664, -3.744133333333333, -3.7499, -3.7556666666666665, -3.761433333333333, -3.7672, -3.7729666666666666, -3.7787333333333333, -3.7845, -3.7902666666666667, -3.796033333333333, -3.8018, -3.8075666666666663, -3.813333333333333, -3.8190999999999997, -3.8248666666666664, -3.830633333333333, -3.8364, -3.8421666666666665, -3.847933333333333, -3.8537, -3.8594666666666666, -3.8652333333333333, -3.8709999999999996, -3.8767666666666667, -3.882533333333333, -3.8882999999999996, -3.8940666666666663, -3.899833333333333, -3.9055999999999997, -3.9113666666666664, -3.917133333333333, -3.9229, -3.9286666666666665, -3.9344333333333332, -3.9402, -3.9459666666666666, -3.9517333333333333, -3.9574999999999996, -3.9632666666666663, -3.969033333333333, -3.9747999999999997, -3.9805666666666664, -3.986333333333333, -3.9920999999999998, -3.9978666666666665, -4.003633333333333, -4.009399999999999, -4.0151666666666666, -4.020933333333333, -4.0267, -4.032466666666666, -4.038233333333333, -4.044, -4.049766666666667, -4.055533333333333, -4.061299999999999, -4.067066666666666, -4.0728333333333335, -4.0786, -4.084366666666666, -4.090133333333333, -4.095899999999999, -4.101666666666667, -4.107433333333333, -4.1132, -4.118966666666666, -4.124733333333333, -4.1305, -4.136266666666667, -4.142033333333333, -4.1478, -4.153566666666666, -4.159333333333333, -4.1651, -4.170866666666666, -4.176633333333333, -4.1823999999999995, -4.188166666666667, -4.193933333333333, -4.1997, -4.205466666666666, -4.211233333333333, -4.217, -4.222766666666667, -4.228533333333333, -4.234299999999999, -4.240066666666666, -4.245833333333333, -4.2516, -4.257366666666666, -4.263133333333333, -4.2688999999999995, -4.274666666666667, -4.280433333333333, -4.2862, -4.291966666666666, -4.297733333333333, -4.3035, -4.309266666666666, -4.315033333333333, -4.320799999999999, -4.3265666666666664, -4.332333333333333, -4.3381, -4.343866666666666, -4.349633333333333, -4.3553999999999995, -4.361166666666667, -4.366933333333333, -4.3727, -4.378466666666666, -4.3842333333333325, -4.39], "Enable Ch"=TRUE, "Hinge Points"=192}, {"Times"=[7000.6, 47596.288, 51000.288], "Voltages"=[2.0, 1.0, 2.5], "Enable Ch"=TRUE, "Hinge Points"=3}, {"Times"=[], "Voltages"=[], "Enable Ch"=TRUE, "Hinge Points"=0}, {"Times"=[], "Voltages"=[], "Enable Ch"=FALSE, "Hinge Points"=0}, {"Times"=[], "Voltages"=[], "Enable Ch"=FALSE, "Hinge Points"=0}, {"Times"=[], "Voltages"=[], "Enable Ch"=FALSE, "Hinge Points"=0}, {"Times"=[], "Voltages"=[], "Enable Ch"=FALSE, "Hinge Points"=0}, {"Times"=[], "Voltages"=[], "Enable Ch"=FALSE, "Hinge Points"=0}, {"Times"=[], "Voltages"=[], "Enable Ch"=FALSE, "Hinge Points"=0}, {"Times"=[], "Voltages"=[], "Enable Ch"=FALSE, "Hinge Points"=0}, {"Times"=[], "Voltages"=[], "Enable Ch"=TRUE, "Hinge Points"=0}] {"Voltages" format="%.2f"; "Times" format="%.2f"}, 2 "Input":i64[][](array[numeric])=array2537x4[10148 elements], 3 "GPIB Input":T1(array[cluster])=[{"Enable"=TRUE, "Abs Start Time"=47001.288, "Module"=31, "String"="Freq 9.8MHz; POW:AMPL -12dBm;", "Array"=["30"]}, {"Enable"=TRUE, "Abs Start Time"=47001.288, "Module"=31, "String"="OUTP:STAT ON;:FM1:DEV 1.0MHz;", "Array"=["30"]}, {"Enable"=TRUE, "Abs Start Time"=47001.288, "Module"=31, "String"=":FM1:STAT ON;", "Array"=["30"]}, {"Enable"=TRUE, "Abs Start Time"=47001.288, "Module"=31, "String"="OUTP ON;", "Array"=["11"]}, {"Enable"=TRUE, "Abs Start Time"=47001.288, "Module"=31, "String"="Freq 6900.9MHz; POW:AMPL 0dbm;:FM1:STAT ON;", "Array"=["19", ""]}, {"Enable"=TRUE, "Abs Start Time"=47001.288, "Module"=31, "String"="OUTP ON;", "Array"=["10", ""]}, {"Enable"=TRUE, "Abs Start Time"=47001.288, "Module"=31, "String"="OUTP:STAT ON;:FM1:DEV 0.6MHz;", "Array"=["19"]}, {"Enable"=TRUE, "Abs Start Time"=48001.288, "Module"=31, "String"="OUTP:STAT OFF;:FM1:STAT OFF;", "Array"=["19"]}, {"Enable"=TRUE, "Abs Start Time"=48001.288, "Module"=31, "String"="OUTP OFF;", "Array"=["10"]}, {"Enable"=TRUE, "Abs Start Time"=48001.288, "Module"=31, "String"="OUTP OFF;", "Array"=["11"]}, {"Enable"=TRUE, "Abs Start Time"=48001.288, "Module"=31, "String"="OUTP:STAT OFF;:FM1:STAT OFF;", "Array"=["30"]}, {"Enable"=TRUE, "Abs Start Time"=50100.288, "Module"=31, "String"="Freq 8038.65MHz; POW:AMPL 8dbm;:FM1:STAT ON;", "Array"=["19", ""]}, {"Enable"=TRUE, "Abs Start Time"=50100.288, "Module"=31, "String"="OUTP:STAT ON;:FM1:DEV 5MHz;", "Array"=["19", ""]}, {"Enable"=TRUE, "Abs Start Time"=51600.288, "Module"=31, "String"="OUTP:STAT OFF;:FM1:STAT OFF;", "Array"=["19", ""]}, {"Enable"=TRUE, "Abs Start Time"=50100.288, "Module"=31, "String"="OUTP ON;", "Array"=["10", ""]}, {"Enable"=TRUE, "Abs Start Time"=51600.288, "Module"=31, "String"="OUTP OFF;", "Array"=["10", ""]}] {"Module" items=["TTL high                                                                                 ", "TTL low                          ", "Camera Strobe                   ", "CMOT", "Defaults                           ", "Fluorescence pulse           ", "IP trap                         ", "Kinetics OD image          ", "Kinetics picture", "Kinetics probe pulse", "MOT light only                ", "MOT off                                   ", "MOT on                         ", "Move cart                      ", "OD image                     ", "Optical pumping          ", "Picture                             ", "Probe Pulse", "Quadrupole trap             ", "IP off", "Utility Module 02           ", "Utility Module 03           ", "Molasses          ", "Utility Module 04     ", "Utility Module 05     ", "Utility Module 06     ", "Utility Module 07     ", "Utility Module 08     ", "Utility Module 09     ", "Utility Module 10     ", "Static DAC", "GPIB"]; "Abs Start Time" format="%.3f"}, 4 "Do this?":bool=TRUE) -> (5 "Static output":T4(array[cluster])=[{"Times"=[6954.0, 7000.1], "Voltages"=[-0.1, -1.0], "Enable Ch"=TRUE, "Hinge Points"=2}, {"Times"=[6944.0, 6994.0, 7000.0], "Voltages"=[-1.0, 2.5, -1.0], "Enable Ch"=TRUE, "Hinge Points"=3}, {"Times"=[6944.0, 6994.0, 7000.0], "Voltages"=[0.0, 0.6, -1.0], "Enable Ch"=TRUE, "Hinge Points"=3}, {"Times"=[6944.0, 6994.0, 7000.0], "Voltages"=[4.0, 0.65, -1.0], "Enable Ch"=TRUE, "Hinge Points"=3}, {"Times"=[6992.0, 7000.6], "Voltages"=[0.0, 2.7], "Enable Ch"=TRUE, "Hinge Points"=2}, {"Times"=[7000.6, 7011.1], "Voltages"=[0.25, 3.0], "Enable Ch"=TRUE, "Hinge Points"=2}, {"Times"=[], "Voltages"=[], "Enable Ch"=TRUE, "Hinge Points"=0}, {"Times"=[48001.288, 48011.488, 48021.688, 48031.888, 48042.088, 48052.288, 48062.488, 48072.688, 48082.888, 48093.088, 48103.288, 48113.488, 48123.688, 48133.888, 48144.088, 48154.288, 48164.488, 48174.688, 48184.888, 48195.088, 48205.288, 48215.488, 48225.688, 48235.888, 48246.088, 48256.288, 48266.488, 48276.688, 48286.888, 48297.088, 48307.288, 48317.488, 48327.688, 48337.888, 48348.088, 48358.288, 48368.488, 48378.688, 48388.888, 48399.088, 48409.288, 48419.488, 48429.688, 48439.888, 48450.088, 48460.288, 48470.488, 48480.688, 48490.888, 48501.088, 48511.288], "Voltages"=[0.0, -0.0052, -0.0104, -0.0156, -0.0208, -0.026, -0.0312, -0.0364, -0.0416, -0.046799999999999994, -0.052, -0.0572, -0.0624, -0.0676, -0.0728, -0.078, -0.0832, -0.08839999999999999, -0.09359999999999999, -0.0988, -0.104, -0.10919999999999999, -0.1144, -0.1196, -0.1248, -0.13, -0.1352, -0.1404, -0.1456, -0.1508, -0.156, -0.16119999999999998, -0.1664, -0.1716, -0.17679999999999998, -0.182, -0.18719999999999998, -0.1924, -0.1976, -0.20279999999999998, -0.208, -0.2132, -0.21839999999999998, -0.2236, -0.2288, -0.23399999999999999, -0.2392, -0.24439999999999998, -0.2496, -0.25479999999999997, -0.26], "Enable Ch"=TRUE, "Hinge Points"=51}, {"Times"=array[1511 elements], "Voltages"=array[1511 elements], "Enable Ch"=TRUE, "Hinge Points"=231}, {"Times"=array[1109 elements], "Voltages"=array[1109 elements], "Enable Ch"=TRUE, "Hinge Points"=85}, {"Times"=array[1613 elements], "Voltages"=array[1613 elements], "Enable Ch"=TRUE, "Hinge Points"=77}, {"Times"=[6944.0, 6994.0, 7000.6], "Voltages"=[0.15, 0.2, 2.5], "Enable Ch"=TRUE, "Hinge Points"=3}, {"Times"=[10850.0, 47200.188, 47200.288, 47200.338, 47200.388, 47200.438, 47200.488, 47200.538, 47200.588, 47200.638, 47200.688, 47200.738, 47200.788, 47200.838, 47200.888, 47200.938, 47200.988, 47201.038, 47201.088, 47201.138, 47201.188, 47201.238, 47201.288, 48501.788, 48001.288, 48003.788, 48006.288, 48008.788, 48011.288, 48013.788, 48016.288, 48018.788, 48021.288, 48023.788, 48026.288, 48028.788, 48031.288, 48033.788, 48036.288, 48038.788, 48041.288, 48043.788, 48046.288, 48048.788, 48051.288, 48053.788, 48056.288, 48058.788, 48061.288, 48063.788, 48066.288, 48068.788, 48071.288, 48073.788, 48076.288, 48078.788, 48081.288, 48083.788, 48086.288, 48088.788, 48091.288, 48093.788, 48096.288, 48098.788, 48101.288, 48103.788, 48106.288, 48108.788, 48111.288, 48113.788, 48116.288, 48118.788, 48121.288, 48123.788, 48126.288, 48128.788, 48131.288, 48133.788, 48136.288, 48138.788, 48141.288, 48143.788, 48146.288, 48148.788, 48151.288, 48153.788, 48156.288, 48158.788, 48161.288, 48163.788, 48166.288, 48168.788, 48171.288, 48173.788, 48176.288, 48178.788, 48181.288, 48183.788, 48186.288, 48188.788, 48191.288, 48193.788, 48196.288, 48198.788, 48201.288, 48203.788, 48206.288, 48208.788, 48211.288, 48213.788, 48216.288, 48218.788, 48221.288, 48223.788, 48226.288, 48228.788, 48231.288, 48233.788, 48236.288, 48238.788, 48241.288, 48243.788, 48246.288, 48248.788, 48251.288, 48253.788, 48256.288, 48258.788, 48261.288, 48263.788, 48266.288, 48268.788, 48271.288, 48273.788, 48276.288, 48278.788, 48281.288, 48283.788, 48286.288, 48288.788, 48291.288, 48293.788, 48296.288, 48298.788, 48301.288, 48303.788, 48306.288, 48308.788, 48311.288, 48313.788, 48316.288, 48318.788, 48321.288, 48323.788, 48326.288, 48328.788, 48331.288, 48333.788, 48336.288, 48338.788, 48341.288, 48343.788, 48346.288, 48348.788, 48351.288, 48353.788, 48356.288, 48358.788, 48361.288, 48363.788, 48366.288, 48368.788, 48371.288, 48373.788, 48376.288, 48378.788, 48381.288, 48383.788, 48386.288, 48388.788, 48391.288, 48393.788, 48396.288, 48398.788, 48401.288, 48403.788, 48406.288, 48408.788, 48411.288, 48413.788, 48416.288, 48418.788, 48421.288, 48423.788, 48426.288, 48428.788, 48431.288, 48433.788, 48436.288, 48438.788, 48441.288, 48443.788, 48446.288, 48448.788, 48451.288, 48453.788, 48456.288, 48458.788, 48461.288, 48463.788, 48466.288, 48468.788, 48471.288, 48473.788, 48476.288, 48478.788, 48481.288, 48483.788, 48486.288, 48488.788, 48491.288, 48493.788, 48496.288, 48498.788, 48501.288], "Voltages"=[0.0, 2.978, 2.978, 2.8241, 2.6702000000000004, 2.5163, 2.3624, 2.2085, 2.0546, 1.9007, 1.7468000000000001, 1.5929000000000002, 1.439, 1.2851000000000001, 1.1312000000000002, 0.9773000000000001, 0.8233999999999999, 0.6695000000000002, 0.5156000000000001, 0.3616999999999999, 0.2078000000000002, 0.05390000000000006, -0.10000000000000009, 0.0, 0.0, 0.00065, 0.0013, 0.00195, 0.0026, 0.00325, 0.0039, 0.00455, 0.0052, 0.005849999999999999, 0.0065, 0.00715, 0.0078, 0.00845, 0.0091, 0.00975, 0.0104, 0.011049999999999999, 0.011699999999999999, 0.01235, 0.013, 0.013649999999999999, 0.0143, 0.01495, 0.0156, 0.01625, 0.0169, 0.01755, 0.0182, 0.01885, 0.0195, 0.020149999999999998, 0.0208, 0.02145, 0.022099999999999998, 0.02275, 0.023399999999999997, 0.02405, 0.0247, 0.025349999999999998, 0.026, 0.02665, 0.027299999999999998, 0.02795, 0.0286, 0.029249999999999998, 0.0299, 0.030549999999999997, 0.0312, 0.031849999999999996, 0.0325, 0.03315, 0.0338, 0.03445, 0.0351, 0.03575, 0.0364, 0.03705, 0.0377, 0.038349999999999995, 0.039, 0.03965, 0.040299999999999996, 0.04095, 0.0416, 0.042249999999999996, 0.0429, 0.04355, 0.044199999999999996, 0.04485, 0.0455, 0.04615, 0.046799999999999994, 0.04745, 0.0481, 0.048749999999999995, 0.0494, 0.05005, 0.050699999999999995, 0.05135, 0.052, 0.052649999999999995, 0.0533, 0.05395, 0.054599999999999996, 0.05525, 0.0559, 0.056549999999999996, 0.0572, 0.05785, 0.058499999999999996, 0.059149999999999994, 0.0598, 0.06045, 0.061099999999999995, 0.06175, 0.0624, 0.06305, 0.06369999999999999, 0.06434999999999999, 0.065, 0.06565, 0.0663, 0.06695, 0.0676, 0.06824999999999999, 0.0689, 0.06955, 0.0702, 0.07085, 0.0715, 0.07214999999999999, 0.0728, 0.07345, 0.0741, 0.07475, 0.0754, 0.07604999999999999, 0.07669999999999999, 0.07735, 0.078, 0.07865, 0.0793, 0.07995, 0.08059999999999999, 0.08125, 0.0819, 0.08255, 0.0832, 0.08385, 0.08449999999999999, 0.08514999999999999, 0.0858, 0.08645, 0.0871, 0.08775, 0.08839999999999999, 0.08904999999999999, 0.0897, 0.09035, 0.091, 0.09165, 0.0923, 0.09294999999999999, 0.09359999999999999, 0.09425, 0.0949, 0.09555, 0.0962, 0.09684999999999999, 0.09749999999999999, 0.09815, 0.0988, 0.09945, 0.1001, 0.10074999999999999, 0.10139999999999999, 0.10205, 0.1027, 0.10335, 0.104, 0.10464999999999999, 0.10529999999999999, 0.10594999999999999, 0.1066, 0.10725, 0.1079, 0.10855, 0.10919999999999999, 0.10984999999999999, 0.1105, 0.11115, 0.1118, 0.11245, 0.11309999999999999, 0.11374999999999999, 0.1144, 0.11505, 0.1157, 0.11635, 0.11699999999999999, 0.11764999999999999, 0.11829999999999999, 0.11895, 0.1196, 0.12025, 0.1209, 0.12154999999999999, 0.12219999999999999, 0.12285, 0.1235, 0.12415, 0.1248, 0.12545, 0.1261, 0.12675, 0.12739999999999999, 0.12805, 0.12869999999999998, 0.12935, 0.13], "Enable Ch"=TRUE, "Hinge Points"=225}, {"Times"=array[705 elements], "Voltages"=array[705 elements], "Enable Ch"=TRUE, "Hinge Points"=193}, {"Times"=[7000.6, 47596.288, 51000.288, 52099.288], "Voltages"=[2.0, 1.0, 2.5, 0.19073], "Enable Ch"=TRUE, "Hinge Points"=4}, {"Times"=array[503 elements], "Voltages"=array[503 elements], "Enable Ch"=TRUE, "Hinge Points"=247}] {"Voltages" format="%.2f"; "Times" format="%.2f"}, 6 "Output":i64[][](array[numeric]), 7 "GPIB Output":T1(array[cluster])=[{"Enable"=TRUE, "Abs Start Time"=47001.288, "Module"=31, "String"="Freq 9.8MHz; POW:AMPL -12dBm;", "Array"=["30"]}, {"Enable"=TRUE, "Abs Start Time"=47001.288, "Module"=31, "String"="OUTP:STAT ON;:FM1:DEV 1.0MHz;", "Array"=["30"]}, {"Enable"=TRUE, "Abs Start Time"=47001.288, "Module"=31, "String"=":FM1:STAT ON;", "Array"=["30"]}, {"Enable"=TRUE, "Abs Start Time"=47001.288, "Module"=31, "String"="OUTP ON;", "Array"=["11"]}, {"Enable"=TRUE, "Abs Start Time"=47001.288, "Module"=31, "String"="Freq 6900.9MHz; POW:AMPL 0dbm;:FM1:STAT ON;", "Array"=["19", ""]}, {"Enable"=TRUE, "Abs Start Time"=47001.288, "Module"=31, "String"="OUTP ON;", "Array"=["10", ""]}, {"Enable"=TRUE, "Abs Start Time"=47001.288, "Module"=31, "String"="OUTP:STAT ON;:FM1:DEV 0.6MHz;", "Array"=["19"]}, {"Enable"=TRUE, "Abs Start Time"=48001.288, "Module"=31, "String"="OUTP:STAT OFF;:FM1:STAT OFF;", "Array"=["19"]}, {"Enable"=TRUE, "Abs Start Time"=48001.288, "Module"=31, "String"="OUTP OFF;", "Array"=["10"]}, {"Enable"=TRUE, "Abs Start Time"=48001.288, "Module"=31, "String"="OUTP OFF;", "Array"=["11"]}, {"Enable"=TRUE, "Abs Start Time"=48001.288, "Module"=31, "String"="OUTP:STAT OFF;:FM1:STAT OFF;", "Array"=["30"]}, {"Enable"=TRUE, "Abs Start Time"=50100.288, "Module"=31, "String"="Freq 8038.65MHz; POW:AMPL 8dbm;:FM1:STAT ON;", "Array"=["19", ""]}, {"Enable"=TRUE, "Abs Start Time"=50100.288, "Module"=31, "String"="OUTP:STAT ON;:FM1:DEV 5MHz;", "Array"=["19", ""]}, {"Enable"=TRUE, "Abs Start Time"=51600.288, "Module"=31, "String"="OUTP:STAT OFF;:FM1:STAT OFF;", "Array"=["19", ""]}, {"Enable"=TRUE, "Abs Start Time"=50100.288, "Module"=31, "String"="OUTP ON;", "Array"=["10", ""]}, {"Enable"=TRUE, "Abs Start Time"=51600.288, "Module"=31, "String"="OUTP OFF;", "Array"=["10", ""]}] {"Module" items=["TTL high                                                                                 ", "TTL low                          ", "Camera Strobe                   ", "CMOT", "Defaults                           ", "Fluorescence pulse           ", "IP trap                         ", "Kinetics OD image          ", "Kinetics picture", "Kinetics probe pulse", "MOT light only                ", "MOT off                                   ", "MOT on                         ", "Move cart                      ", "OD image                     ", "Optical pumping          ", "Picture                             ", "Probe Pulse", "Quadrupole trap             ", "IP off", "Utility Module 02           ", "Utility Module 03           ", "Molasses          ", "Utility Module 04     ", "Utility Module 05     ", "Utility Module 06     ", "Utility Module 07     ", "Utility Module 08     ", "Utility Module 09     ", "Utility Module 10     ", "Static DAC", "GPIB"]; "Abs Start Time" format="%.3f"})   [LabVIEW 2017]
uses:
  globals/Modules global.vi
panel:
  in  "Read/Write":bool
  in  "Do Write/Read":bool
  in  "Manual Array":T2(array[cluster])=[{"Time2 (ms)"="290.000", "Port2"=2, "Line2"=0, "Comments2"="Bias Field reference change to PC Input (1,0,0)", "Value2"=TRUE, "Enable2"=TRUE, "DAC value"="0"}, {"Time2 (ms)"="290.000", "Port2"=2, "Line2"=1, "Comments2"="", "Value2"=FALSE, "Enable2"=TRUE, "DAC value"="0"}, {"Time2 (ms)"="290.000", "Port2"=2, "Line2"=2, "Comments2"="", "Value2"=FALSE, "Enable2"=TRUE, "DAC value"="0"}, {"Time2 (ms)"="290.500", "Port2"=2, "Line2"=3, "Comments2"="Bias field servo integrator OFF", "Value2"=FALSE, "Enable2"=TRUE, "DAC value"="0"}, {"Time2 (ms)"="300.050", "Port2"=2, "Line2"=3, "Comments2"="Bias field servo integrator ON", "Value2"=TRUE, "Enable2"=TRUE, "DAC value"="0"}, {"Time2 (ms)"="602.000", "Port2"=4, "Line2"=9, "Comments2"="Turn OFF Cart QT", "Value2"=TRUE, "Enable2"=TRUE, "DAC value"="5"}, {"Time2 (ms)"="601.950", "Port2"=2, "Line2"=5, "Comments2"="MOT QT integrator OFF", "Value2"=TRUE, "Enable2"=TRUE, "DAC value"="0"}, {"Time2 (ms)"="603.000", "Port2"=2, "Line2"=5, "Comments2"="MOT QT integrator ON", "Value2"=FALSE, "Enable2"=TRUE, "DAC value"="0"}, {"Time2 (ms)"="0.000", "Port2"=2, "Line2"=7, "Comments2"="Turn off MOT shim coil L/R", "Value2"=FALSE, "Enable2"=TRUE, "DAC value"="0"}, {"Time2 (ms)"="0.000", "Port2"=2, "Line2"=8, "Comments2"="Turn off MOT shim coil U/D", "Value2"=FALSE, "Enable2"=TRUE, "DAC value"="0"}, {"Time2 (ms)"="0.000", "Port2"=2, "Line2"=9, "Comments2"="Turn off MOT shim coil F/B", "Value2"=FALSE, "Enable2"=TRUE, "DAC value"="0"}, {"Time2 (ms)"="1000.000", "Port2"=2, "Line2"=10, "Comments2"="Turn on Sci shim coil L/R", "Value2"=TRUE, "Enable2"=TRUE, "DAC value"="0"}, {"Time2 (ms)"="1000.000", "Port2"=2, "Line2"=11, "Comments2"="Turn on Sci shim coil U/D", "Value2"=TRUE, "Enable2"=TRUE, "DAC value"="0"}, {"Time2 (ms)"="1000.000", "Port2"=2, "Line2"=12, "Comments2"="Turn on Sci shim coil F/B", "Value2"=TRUE, "Enable2"=TRUE, "DAC value"="0"}, {"Time2 (ms)"="1000.000", "Port2"=4, "Line2"=13, "Comments2"="Sci shim coil L/R compensate bg B-field", "Value2"=FALSE, "Enable2"=TRUE, "DAC value"="0"}, {"Time2 (ms)"="1000.000", "Port2"=4, "Line2"=14, "Comments2"="Sci shim coil U/D compensate bg B-field", "Value2"=FALSE, "Enable2"=TRUE, "DAC value"="0.19073"}, {"Time2 (ms)"="1000.000", "Port2"=4, "Line2"=15, "Comments2"="Sci shim coil F/B compensate bg B-field", "Value2"=FALSE, "Enable2"=TRUE, "DAC value"="0.21965"}, {"Time2 (ms)"="1050.000", "Port2"=4, "Line2"=14, "Comments2"="previous set: 0.1557", "Value2"=FALSE, "Enable2"=FALSE, "DAC value"="1"}, {"Time2 (ms)"="1050.000", "Port2"=4, "Line2"=15, "Comments2"="shift QT center", "Value2"=FALSE, "Enable2"=TRUE, "DAC value"="2.6"}, {"Time2 (ms)"="1050.000", "Port2"=4, "Line2"=13, "Comments2"="shift QT center", "Value2"=FALSE, "Enable2"=FALSE, "DAC value"="5"}, {"Time2 (ms)"="10000.000", "Port2"=0, "Line2"=0, "Comments2"="", "Value2"=TRUE, "Enable2"=FALSE, "DAC value"="0"}, {"Time2 (ms)"="10001.000", "Port2"=0, "Line2"=0, "Comments2"="", "Value2"=FALSE, "Enable2"=FALSE, "DAC value"="0"}, {"Time2 (ms)"="0.000", "Port2"=3, "Line2"=11, "Comments2"="790 shutter ON", "Value2"=TRUE, "Enable2"=FALSE, "DAC value"="0"}, {"Time2 (ms)"="10000.000", "Port2"=3, "Line2"=11, "Comments2"="790 AOM ON", "Value2"=TRUE, "Enable2"=FALSE, "DAC value"="0"}, {"Time2 (ms)"="11000.000", "Port2"=3, "Line2"=11, "Comments2"="790 AOM OFF", "Value2"=FALSE, "Enable2"=FALSE, "DAC value"="0"}] {"Line2" items=["0", "1", "2", "3", "4", "5", "6", "7", "8", "9", "10", "11", "12", "13", "14", "15", "16", "17", "18", "19", "20", "21", "22", "23", "24", "25", "26", "27", "28", "29", "30", "31"]; "Port2" items=["A", "B", "C", "D", "DAC", "GPIB"]}
  in  "filename":string="Loading sci QT"
  in  "Static DAC Linear Ramps":T3(array[cluster])=[{"Write Ramp?"=TRUE, "DAC Channel"=8, "Ramp begin"="0.000", "Ramp end"="300.000", "start value"="2.400", "end value"="1.200", "steps"="500"}, {"Write Ramp?"=TRUE, "DAC Channel"=9, "Ramp begin"="0.000", "Ramp end"="300.000", "start value"="-4.400", "end value"="-2.100", "steps"="500"}, {"Write Ramp?"=TRUE, "DAC Channel"=10, "Ramp begin"="301.000", "Ramp end"="601.000", "start value"="0.000", "end value"="-3.600", "steps"="500"}, {"Write Ramp?"=TRUE, "DAC Channel"=9, "Ramp begin"="301.000", "Ramp end"="601.000", "start value"="-2.100", "end value"="0.000", "steps"="500"}, {"Write Ramp?"=TRUE, "DAC Channel"=8, "Ramp begin"="650.000", "Ramp end"="950.000", "start value"="1.200", "end value"="2.000", "steps"="500"}, {"Write Ramp?"=TRUE, "DAC Channel"=10, "Ramp begin"="650.000", "Ramp end"="950.000", "start value"="-3.600", "end value"="-6.000", "steps"="500"}, {"Write Ramp?"=TRUE, "DAC Channel"=8, "Ramp begin"="8250.00", "Ramp end"="10000.0", "start value"="2.000", "end value"="0.7000", "steps"="500"}, {"Write Ramp?"=TRUE, "DAC Channel"=10, "Ramp begin"="8250.00", "Ramp end"="10000.0", "start value"="-6.000", "end value"="-2.100", "steps"="500"}, {"Write Ramp?"=TRUE, "DAC Channel"=15, "Ramp begin"="8250.00", "Ramp end"="10000.0", "start value"="2.600", "end value"="1.022", "steps"="500"}] {"DAC Channel" items=["0", "1", "2", "3", "4", "5", "6", "7", "8", "9", "10", "11", "12", "13", "14", "15", "16", "17", "18", "19", "20", "21", "22", "23"]}
  # "Time                   Port        Line       Value  Enable  DAC voltage  Comments"
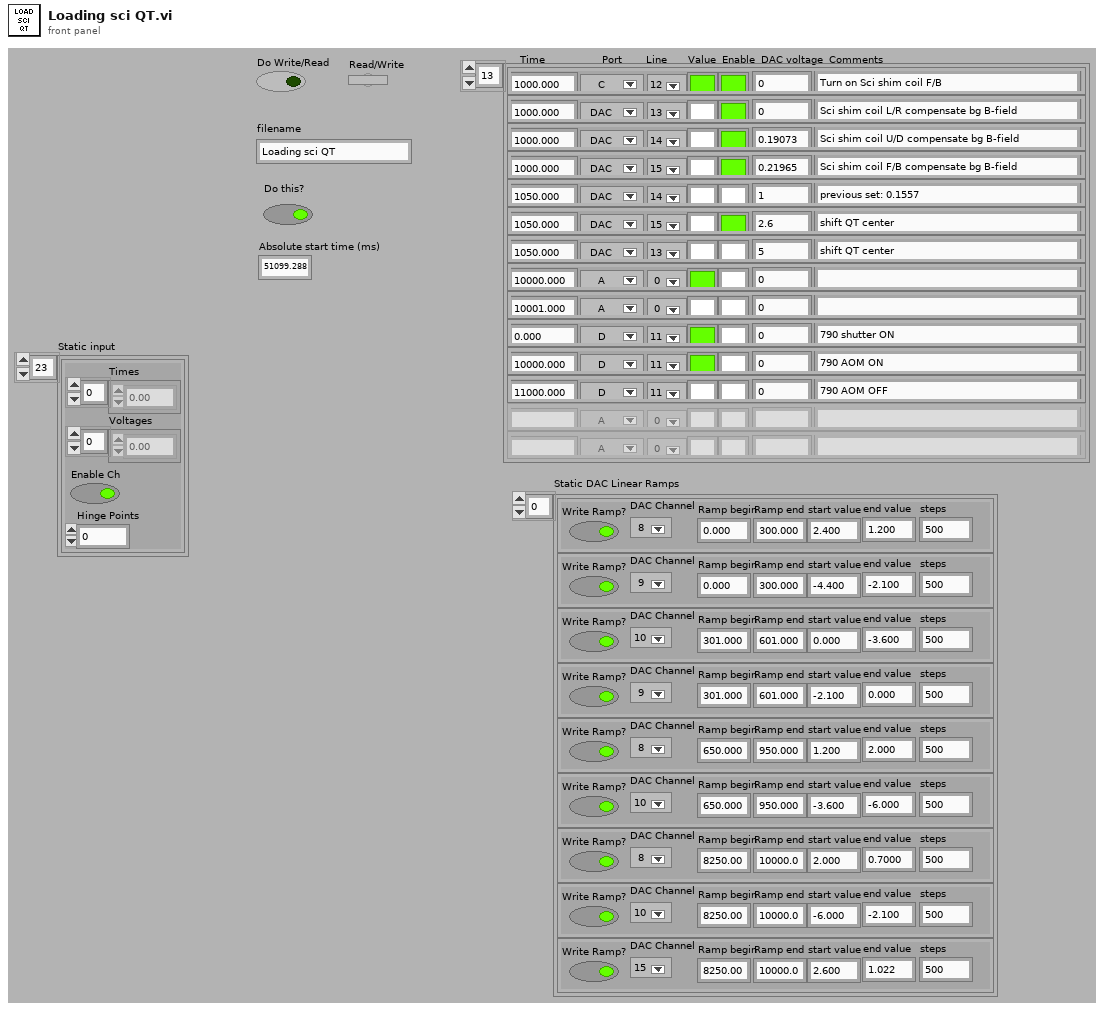
[diagram p1: front panel]
types:
  T1 = cluster{"Enable":bool, "Abs Start Time":dbl, "Module":u16, "String":string, "Array":string[]}[]
  T2 = cluster{"Time2 (ms)":string, "Port2":u16, "Line2":u16, "Comments2":string, "Value2":bool, "Enable2":bool, "DAC value":string}[]
  T3 = cluster{"Write Ramp?":bool, "DAC Channel":i16, "Ramp begin":string, "Ramp end":string, "start value":string, "end value":string, "steps":string}[]
  T4 = cluster{"Times":dbl[], "Voltages":dbl[], "Enable Ch":bool, "Hinge Points":u8}[]
  T5 = cluster{"Manual Array":cluster{"Time2 (ms)":dbl, "Port2":u16, "Line2":u16, "Comments2":string, "Value2":bool, "Enable2":bool, "DAC value":dbl}[], "Static DAC Linear Ramps":cluster{"Write Ramp?":bool, "DAC Channel":i16, "Ramp begin":dbl, "Ramp end":dbl, "start value":dbl, "end value":dbl, "steps":i16}[]}
  T6 = cluster{"Time2 (ms)":dbl, "Port2":u16, "Line2":u16, "Comments2":string, "Value2":bool, "Enable2":bool, "DAC value":dbl}[]
  T7 = cluster{"Write Ramp?":bool, "DAC Channel":i16, "Ramp begin":dbl, "Ramp end":dbl, "start value":dbl, "end value":dbl, "steps":i16}[]
  T8 = cluster{"Time2 (ms)":string, "Port2":u16, "Line2":u16, "Comments2":string, "Value2":bool, "Enable2":bool, "DAC value":string}
  T9 = cluster{"Write Ramp?":bool, "DAC Channel":i16, "Ramp begin":string, "Ramp end":string, "start value":string, "end value":string, "steps":string}
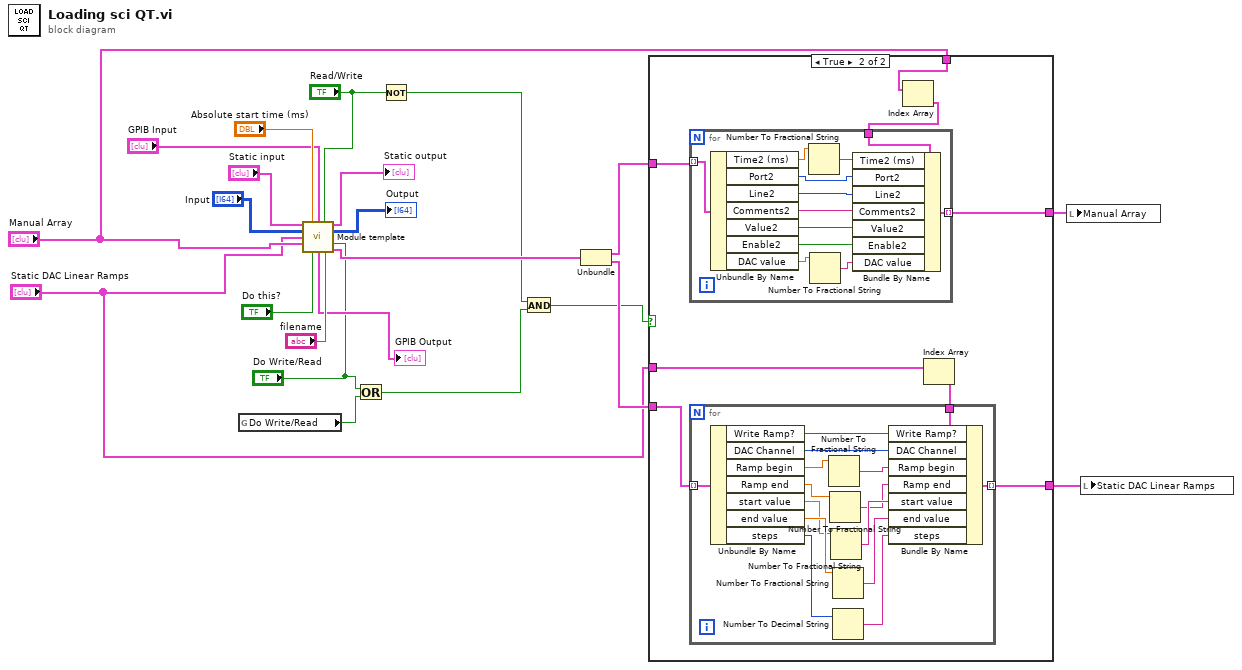
[diagram p0: block diagram]
diagram:
  n1 = global read "Modules global.vi" "Do Write/Read"() -> (w8:bool)
  n2 = call "Module template.vi"("Static input"="Static input", "Absolute start time (ms)"="Absolute start time (ms)", "GPIB Input"="GPIB Input", "Read/Write"="Read/Write", "Input"="Input", "Static DAC Linear Ramps"="Static DAC Linear Ramps", "Manual Array"="Manual Array", "Do Write/Read"="Do Write/Read", "Do this?"="Do this?", "filename"="filename") -> ("Static output"=→"Static output":T4, "Output"=→"Output":i64[][], "GPIB Output"=→"GPIB Output":T1, "Saved Cluster"=w16:T5)  [unwired: 2 in]
  n3 = Or(x="Do Write/Read", y=w8) -> (x .or. y?=w5:bool)
  n4 = Not(x="Read/Write") -> (.not. x?=w6:bool)
  n5 = And(x=w6, y=w5) -> (x .and. y?=w4:bool)
  n6 = Unbundle(w16) -> ("Manual Array"=w11:T6, "Static DAC Linear Ramps"=w10:T7)
  n7 = case shown="True" w4 {
    tunnel: w11 -> [_ w32]
    tunnel: w10 -> [_ w31]
    tunnel: "Manual Array" -> [w23 w30]
    tunnel: "Static DAC Linear Ramps" -> [w24 w28]
    tunnel: [w23 w26] -> w2
    tunnel: [w24 w25] -> w1
    frame False {
    }
    frame True {
      n8 = Index Array(array=w30) -> (element=w29:T8)  [unwired: 1 in]
      n9 = for {
        tunnel: w32 -> [w59] mode=indexing
        tunnel: w29 -> [w58]
        tunnel: [w48] -> w26 mode=indexing
        n10 = Unbundle By Name(w59) -> ("Time2 (ms)"=w51:dbl, "Port2"=w56:u16, "Line2"=w55:u16, "Comments2"=w54:string, "Value2"=w53:bool, "Enable2"=w52:bool, "DAC value"=w50:dbl)
        n11 = Number To Fractional String(number=w51) -> (F-format string=w57:string)  [unwired: 3 in]
        n12 = Number To Fractional String(number=w50) -> (F-format string=w49:string)  [unwired: 3 in]
        n13 = Bundle By Name(cluster=w58, "Time2 (ms)"=w57, "Port2"=w56, "Line2"=w55, "Comments2"=w54, "Value2"=w53, "Enable2"=w52, "DAC value"=w49) -> (w48:T8)
      }
      n14 = Index Array(array=w28) -> (element=w27:T9)  [unwired: 1 in]
      n15 = for {
        tunnel: w31 -> [w47] mode=indexing
        tunnel: w27 -> [w46]
        tunnel: [w33] -> w25 mode=indexing
        n16 = Unbundle By Name(w47) -> ("Write Ramp?"=w45:bool, "DAC Channel"=w44:i16, "Ramp begin"=w34:dbl, "Ramp end"=w37:dbl, "start value"=w39:dbl, "end value"=w41:dbl, "steps"=w43:i16)
        n17 = Number To Fractional String(number=w34) -> (F-format string=w35:string)  [unwired: 3 in]
        n18 = Number To Fractional String(number=w37) -> (F-format string=w36:string)  [unwired: 3 in]
        n19 = Number To Fractional String(number=w39) -> (F-format string=w38:string)  [unwired: 3 in]
        n20 = Number To Fractional String(number=w41) -> (F-format string=w40:string)  [unwired: 3 in]
        n21 = Number To Decimal String(number=w43) -> (decimal integer string=w42:string)  [unwired: 1 in]
        n22 = Bundle By Name(cluster=w46, "Write Ramp?"=w45, "DAC Channel"=w44, "Ramp begin"=w35, "Ramp end"=w36, "start value"=w38, "end value"=w40, "steps"=w42) -> (w33:T9)
      }
    }
  }
  n23 = local write "Manual Array"(w2) -> ()
  n24 = local write "Static DAC Linear Ramps"(w1) -> ()
